vi "LetreroCambios.vi"() -> ()   [LabVIEW 2015]
panel:
  in  "Tab Control":enum32{"Controles", "Letrero"}(tab)
  out "Cambios\nRealizados":dbl
  in  "Cambios\nDeseados":dbl
  in  "Control de\nVelocidad":dbl(slide) scale=0.0..20.0
  in  "Introducir Texto":string
  in  "OK Button":bool
  out "Letrero":string
  # "Más\nLento"
  # "Más\nRapido"
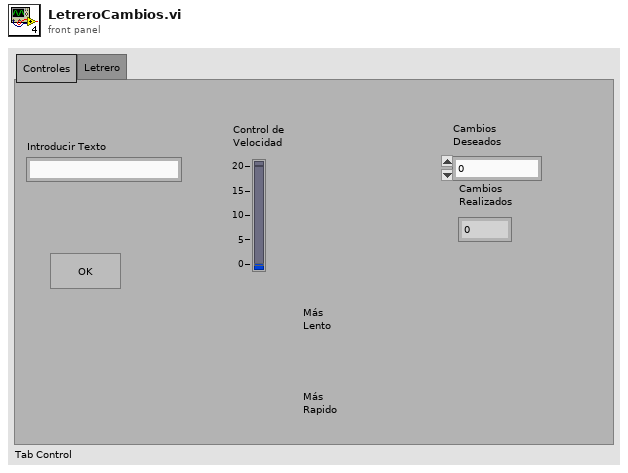
[diagram p1: front panel]
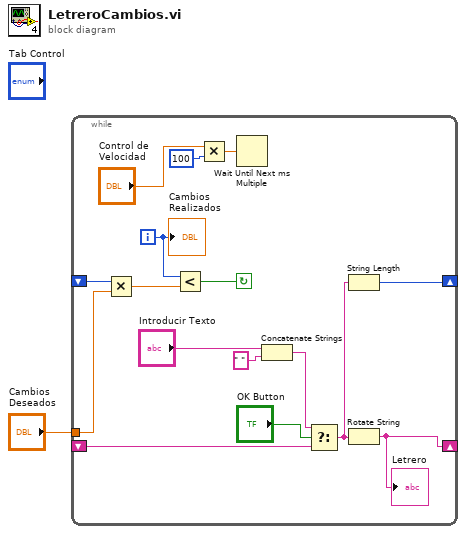
[diagram p0: block diagram]
diagram:
  n1 = while {
    shift-right: [w11] -> _
    shift-left: _ -> [w12]
    shift-right: [w3] -> _
    shift-left: _ -> [w4]
    tunnel: "Cambios\nDeseados" -> [w10]
    i -> [w2]
    stop <- w8 continue-if-true
    n2 = Multiply(x=w4, y=w10) -> (x*y=w9:dbl)
    n3 = Less?(x=w2, y=w9) -> (x < y?=w8:bool)
    n4 = Multiply(x="Control de\nVelocidad", y=100) -> (x*y=w15:dbl)
    n5 = Wait Until Next ms Multiple(millisecond multiple=w15) -> ()  [unwired: 1 out]
    n6 = Concatenate Strings("Introducir Texto", " " ("string")) -> (w5:string)
    n7 = Select(t=w5, s="OK Button", f=w12) -> (s? t:f=w13:string)
    n8 = String Length(string=w13) -> (length=w3:i32)
    n9 = Rotate String(1:w13) -> (0:w11:string)
    "Letrero" <- w11
    "Cambios\nRealizados" <- w2
  }
